vi "Latch.vi"(0 "Input":bool) -> (7 "Output":bool)   [LabVIEW 2012]
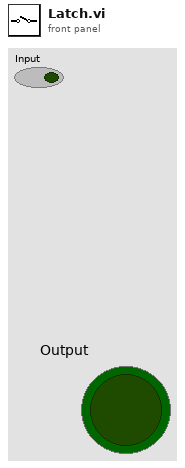
[diagram p1: front panel]
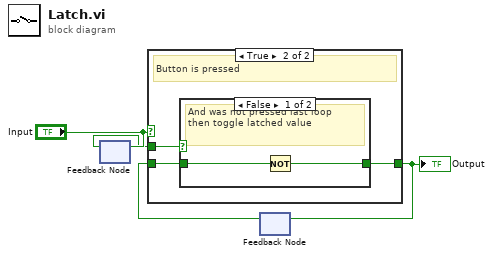
[diagram p0: block diagram]
diagram:
  n1 = feedback-in #1("Input") -> ()
  n2 = feedback #1() -> (w3:bool)  [unwired: 1 in]
  n3 = feedback #2() -> (w1:bool)  [unwired: 1 in]
  n4 = case shown="True" "Input" {
    tunnel: w3 -> [_ w8]
    tunnel: w1 -> [w5 w7]
    tunnel: [w5 w6] -> w2
    frame False {
      # "Button is not pressed"
    }
    frame True {
      # "Button is pressed"
      n5 = case shown="False" w8 {
        tunnel: w7 -> [w9 w11]
        tunnel: [w10 w11] -> w6
        frame False {
          # "And was not pressed last loop\nthen toggle latched value"
          n6 = Not(x=w9) -> (.not. x?=w10:bool)
        }
        frame True {
          # "And was pressed last loop\nthen hold current latched value"
        }
      }
    }
  }
  "Output" <- w2
  n7 = feedback-in #2(w2) -> ()
